vi "Query All Channels.vi"(6 "timeout (ms)":i32=5000, 8 "error in":errorcluster, 10 "Channel Filter":T4, 11 "gRPC ID in":T5) -> (0 "error out":errorcluster, 2 "channels":T1[](array[typedef]) {"custom_config" format="%.0x"}, 3 "gRPC ID out":T5)   [LabVIEW 2021, in "CIFManagerClientWrapper.lvlib"]
uses:
  <vilib>/gRPC/LabVIEW gRPC Library/Shared/grpcId.ctl
  CIFManagerClientWrapper.lvlib
  CIF_Manager_client/CIF_Manager_client.lvlib
  <vilib>/gRPC/LabVIEW gRPC Library/grpc-lvsupport-release.lvlib
  CIF_Manager_client/RPC Messages/cif_channelcore_Direction.ctl
  CIF_Manager_client/RPC Messages/cif_channelcore_ChannelFilter.ctl
  CIF_Manager_client/RPC Messages/cif_channelcore_PATTERN.ctl
  CIF_Manager_client/RPC Messages/cif_channelcore_Channel.ctl
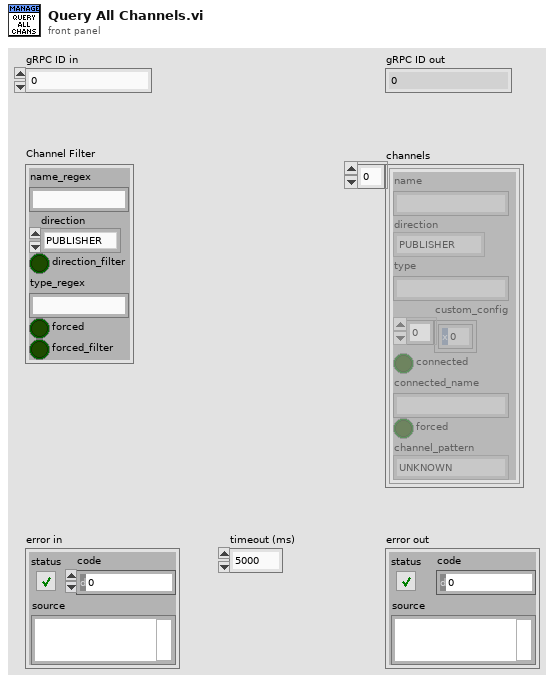
[diagram p1: front panel]
types:
  T1 = typedef "CIF_Manager_client.lvlib/cif_channelcore_Channel.ctl" = cluster{"name":string, "direction":T2, "type":string, "custom_config":u8[], "connected":bool, "connected_name":string, "forced":bool, "channel_pattern":T3}
  T2 = typedef "CIF_Manager_client.lvlib/cif_channelcore_Direction.ctl" = enum32{"PUBLISHER", "SUBSCRIBER"}
  T3 = typedef "CIF_Manager_client.lvlib/cif_channelcore_PATTERN.ctl" = enum32{"UNKNOWN", "TAG", "FIFO", "MULTIFIFO", "BACKPRESSUREFIFO"}
  T4 = typedef "CIF_Manager_client.lvlib/cif_channelcore_ChannelFilter.ctl" = cluster{"name_regex":string, "direction":T2, "direction_filter":bool, "type_regex":string, "forced":bool, "forced_filter":bool}
  T5 = typedef "grpc-lvsupport-release.lvlib/grpcId.ctl" = u64
  T6 = typedef "CIF_Manager_client.lvlib/cif_channelcore_Channels.ctl" = cluster{"channels":T1[]}
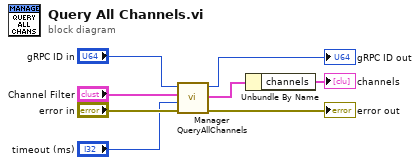
[diagram p0: block diagram]
diagram:
  n1 = call "Manager QueryAllChannels.vi"("error in"="error in", "timeout (ms)"="timeout (ms)", "Request Data"="Channel Filter", "gRPC ID"="gRPC ID in") -> ("error out"=→"error out":errorcluster, "Response Data"=w4:T6, "gRPC ID out"=→"gRPC ID out":T5)  [unwired: 5 in]
  n2 = Unbundle By Name(w4) -> ("channels"=→"channels":T1[])
